vi "UpdateCurvePar.vi"(8 "error in (no error)":errorcluster caption="entrée d'erreur (pas d'erreur)", 10 "PlotChange":T1, 11 "Interface en entrée":refnum<class "Interface.lvclass"> caption="DNL_LabVIEW Object in") -> (0 "error out":errorcluster caption="sortie d'erreur", 3 "Interface en sortie":refnum<class "Interface.lvclass"> caption="DNL_LabVIEW Object out")   [LabVIEW 2019, in "Interface.lvclass"]
uses:
  Interface.lvclass
  PlotChange.ctl
  Interface.lvclass/Interface.ctl
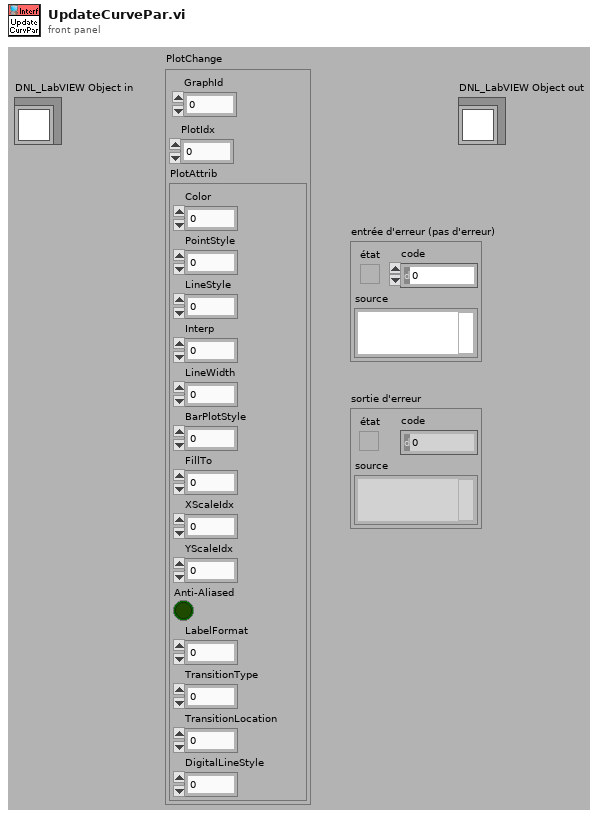
[diagram p1: front panel]
types:
  T1 = typedef "PlotChange.ctl" = cluster{"PlotIdx":i32, "PlotAttrib":cluster{"Color":u32, "PointStyle":u8, "LineStyle":u8, "Interp":u8, "LineWidth":u8, "BarPlotStyle":u8, "FillTo":i16, "XScaleIdx":u32, "YScaleIdx":u32, "Anti-Aliased":bool, "LabelFormat":u8, "TransitionType":u8, "TransitionLocation":u8, "DigitalLineStyle":u8}, "GraphId":i32}
  T2 = cluster{"Color":u32, "PointStyle":u8, "LineStyle":u8, "Interp":u8, "LineWidth":u8, "BarPlotStyle":u8, "FillTo":i16, "XScaleIdx":u32, "YScaleIdx":u32, "Anti-Aliased":bool, "LabelFormat":u8, "TransitionType":u8, "TransitionLocation":u8, "DigitalLineStyle":u8}
  T3 = typedef "Interface.lvclass/CurveSetup.ctl" = cluster{"CurveName":string, "YParam":string, "XParam":string, "ZParam ":string, "GroupName":string, "LinWdth":u8, "PntCol":u32, "LinCol":u32, "LablFor":u8, "XScale":u32, "YScale":u32, "Interpol":u8, "DisplayName":string, "FillType":i16, "LineStyle":u8, "PntStyle":u8, "BarTyp":u8, "GraphIndex":i32, "Visible":bool, "XScaleName":string, "YScaleName":string, "XYGraph_Ref":refnum<vi>, "Data Only":bool, "DataQ Ref":refnum<queue>, "XParQ Ref":refnum<queue>, "XParamInd":i32, "ScanInd":i32}
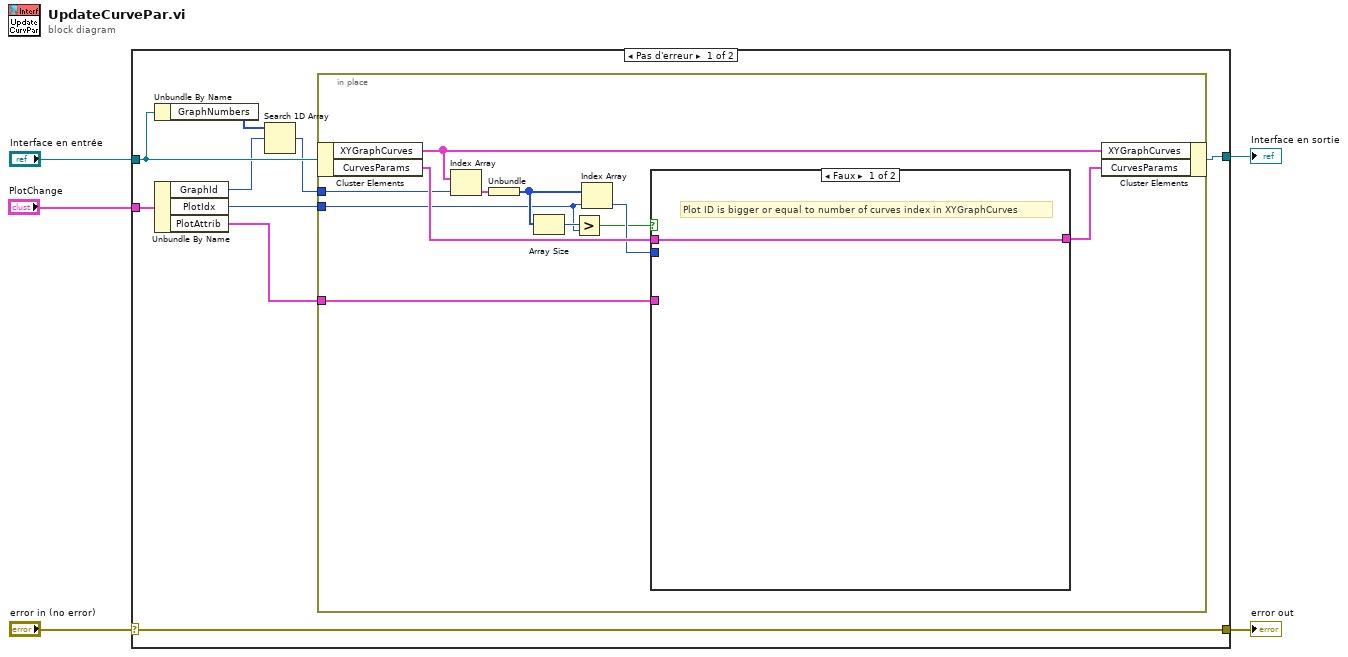
[diagram p0: block diagram]
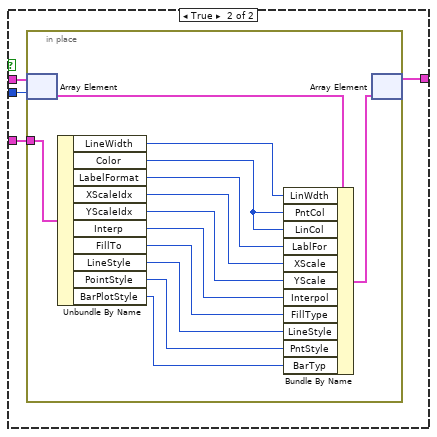
[diagram p2: hidden frame]
diagram:
  n1 = case shown="Pas d'erreur" "error in (no error)" {
    selector: "error in (no error)" -> [w14 w45]
    tunnel: [w14 w45] -> w4
    tunnel: [w13 w44] -> w2
    tunnel: "Interface en entrée" -> [w9 w44]
    tunnel: "PlotChange" -> [w12 _]
    frame No Error {
      n2 = Unbundle By Name(w9) -> ("GraphNumbers"=w8:i32[])
      n3 = Unbundle By Name(w12) -> ("GraphId"=w7:i32, "PlotIdx"=w11:i32, "PlotAttrib"=w10:T2)
      n4 = Search 1D Array(1D array=w8, element=w7) -> (index of element=w6:i32)  [unwired: 1 in]
      n5 = in-place {
        in-place-border: w11 -> [w17]
        in-place-border: w10 -> [w20]
        in-place-border: w6 -> [w15]
        n6 = in-place-cluster #1(w9) -> ("XYGraphCurves"=w24:cluster{"Tableau":i32[]}[], "CurvesParams"=w23:T3[])
        n7 = Index Array(array=w24, index=w15) -> (element=w25:cluster{"Tableau":i32[]})
        n8 = Unbundle(w25) -> ("Tableau"=w19:i32[])
        n9 = Array Size(array=w19) -> (size(s)=w18:i32)
        n10 = Greater?(x=w18, y=w17) -> (0:w16:bool)
        n11 = Index Array(array=w19, index=w17) -> (element=w22:i32)
        n12 = case shown="Faux" w16 {
          tunnel: w23 -> [w26 w30]
          tunnel: w22 -> [_ w29]
          tunnel: [w26 w28] -> w21
          tunnel: w20 -> [_ w27]
          frame False {
            # "Plot ID is bigger or equal to number of curves index in XYGraphCurves"
          }
          frame True {
            n13 = in-place {
              in-place-border: w27 -> [w41]
              n14 = in-place-array #2(w30, w29) -> (w43:T3)
              n15 = Unbundle By Name(w41) -> ("LineWidth"=w39:u8, "Color"=w40:u32, "LabelFormat"=w38:u8, "XScaleIdx"=w37:u32, "YScaleIdx"=w36:u32, "Interp"=w35:u8, "FillTo"=w34:i16, "LineStyle"=w33:u8, "PointStyle"=w32:u8, "BarPlotStyle"=w31:u8)
              n16 = Bundle By Name(cluster=w43, "LinWdth"=w39, "PntCol"=w40, "LinCol"=w40, "LablFor"=w38, "XScale"=w37, "YScale"=w36, "Interpol"=w35, "FillType"=w34, "LineStyle"=w33, "PntStyle"=w32, "BarTyp"=w31) -> (w42:T3)
              n17 = in-place-array #2(w42) -> (w28:T3[])  [unwired: 1 out]
            }
          }
        }
        n18 = in-place-cluster #1("XYGraphCurves"=w24, "CurvesParams"=w21) -> (w13:refnum<class "Interface.lvclass">)
      }
    }
    frame Error {
    }
  }
  "error out" <- w4
  "Interface en sortie" <- w2
